vi "Match Initiate Upload Response.vi"(8 "error in":errorcluster, 10 "Frame Data":u8[](array[numeric]), 11 "SDO Transfer in":refnum<class "SDO Transfer.lvclass">) -> (0 "error out":errorcluster, 1 "SDO Result":T1={"Success"=FALSE, "SDO abort code"={"Null"=FALSE, "Value"=0}, "Data"={"Null"=TRUE, "Data"=[]}} {"SDO abort code"."Value" items=["Toggle bit not allowed"=84082688, "SDO protocol timed out"=84148224, "Client/server command specifier not valid or unknown"=84148225, "Invalid block size (block mode only)"=84148226, "Invalid sequence number (block mode only)"=84148227, "CRC error (block mode only)"=84148228, "Out of memory"=84148229, "Attempt to read a write only object"=100728833, "Attempt to write a read only object"=100728834, "Object does not exist in the object dictionary"=100794368, "Object cannot be mapped to the PDO"=100925505, "The number and length of the objects to be mapped would exceed PDO length"=100925506, "General parameter incompatibility reason"=100925507, "General internal incompatibility in the device"=100925511, "Access failed due to an hardware error"=101056512, "Data type does not match, length of service parameter does not match"=101122064, "Data type does not match, length of service parameter too high"=101122066, "Data type does not match, length of service parameter too low"=101122067, "Sub-index does not exist"=101253137, "Invalid value for parameter (download only)"=101253168, "Value of parameter written too high (download only)"=101253169, "Value of parameter written too low (download only)"=101253170, "Maximum value is less than minimum value"=101253174, "Resource not available: SDO connection"=101318691, "General error"=134217728, "Data cannot be transferred or stored to the application"=134217760, "Data cannot be transferred or stored to the application because of local control"=134217761, "Data cannot be transferred or stored to the application because of the present device stable"=134217762, "Object dictionary dynamic generation fails or no object dictionary is present (e.g. object dictionary is generated from file and generation fails because of an file error)"=134217763, "No data available"=134217764]; "Data"."Data" format="%02x"}, 2 "Match":bool, 3 "SDO Transfer out":refnum<class "SDO Transfer.lvclass">)   [LabVIEW 2020, in "CANopen.lvlib" / "SDO Manager.lvlib" / "Upload Transfer.lvclass"]
uses:
  Upload Transfer.lvclass
  SDO Transfer/SDO Transfer.lvclass
  Segmented Upload Transfer/Segmented Upload Transfer.lvclass
  HAL/Source/Interfaces/ICommunicate/ICommunicate.lvclass
  Upload Transfer.lvclass/Upload Transfer.ctl
  D:/git/CANopen-LabVIEW/source/SDO Manager/SDO Manager/SDO Transfer/SDO Transfer.lvclass
  D:/git/CANopen-LabVIEW/source/Response Matcher/IResponse/IMatch Response.lvclass
  D:/git/CANopen-LabVIEW/source/SDO Manager/SDO Manager/Segmented Upload Transfer/Segmented Upload Transfer.lvclass
  SDO Transfer/SDO abort code.ctl
  Typedefs/SDO Result.ctl
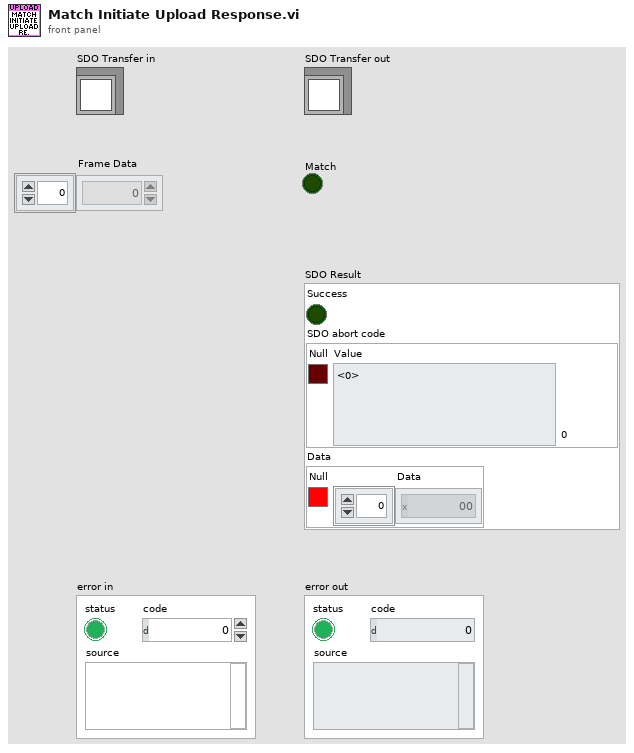
[diagram p1: front panel]
types:
  T1 = typedef "CANopen.lvlib/SDO Manager.lvlib/SDO Transfer.lvclass/SDO Result.ctl" = cluster{"Success":bool, "SDO abort code":cluster{"Null":bool, "Value":T2}, "Data":cluster{"Null":bool, "Data":u8[]}}
  T2 = typedef "CANopen.lvlib/SDO Manager.lvlib/SDO Transfer.lvclass/SDO abort code.ctl" = u32
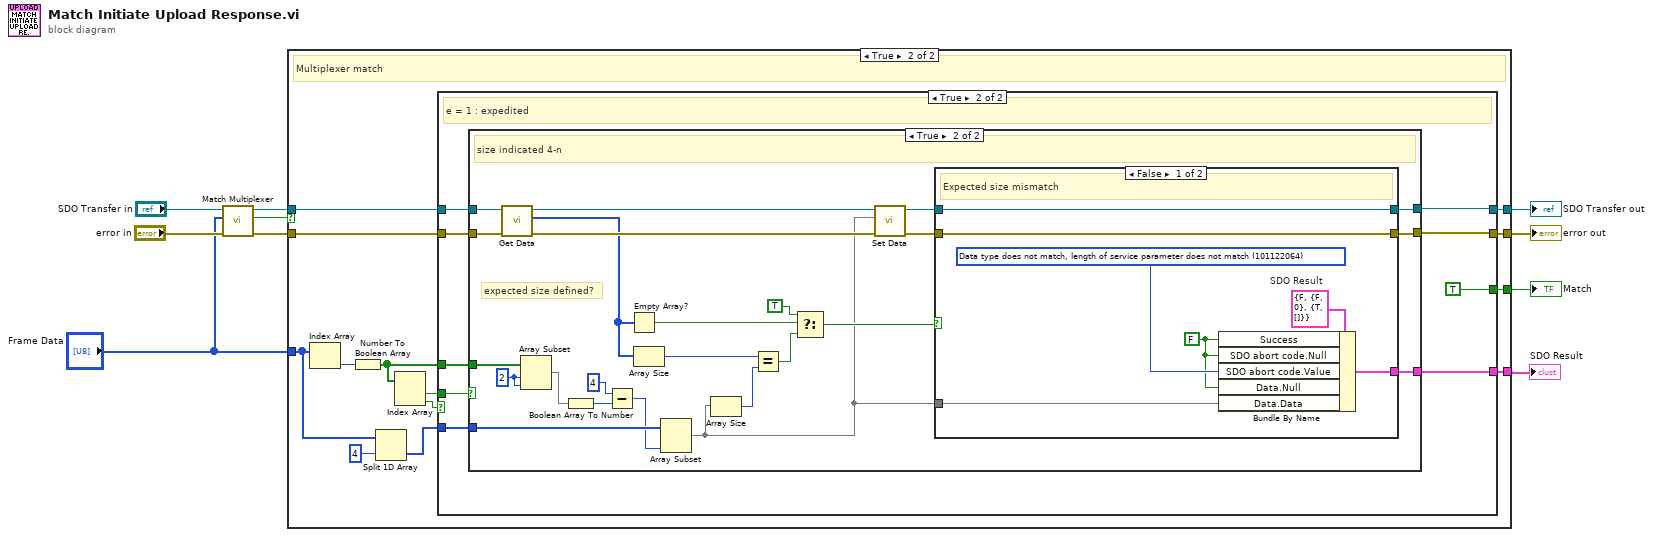
[diagram p0: block diagram]
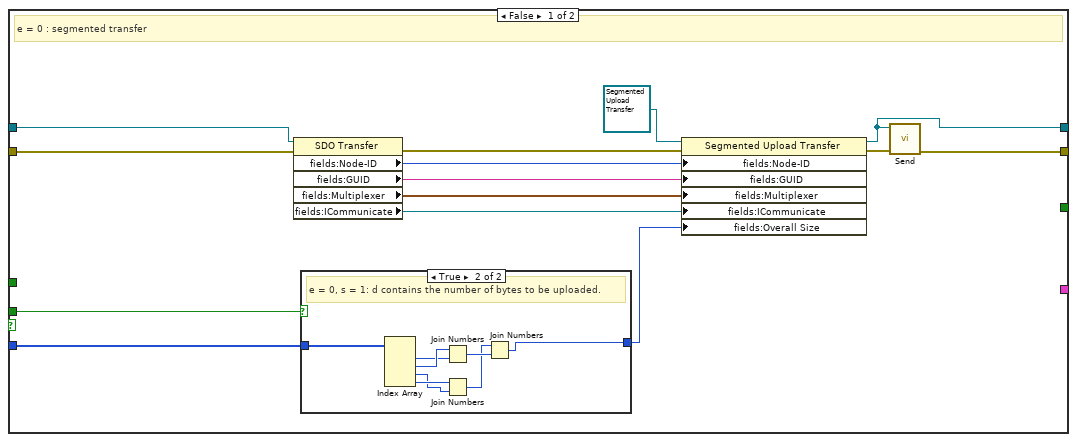
[diagram p3: hidden frame]
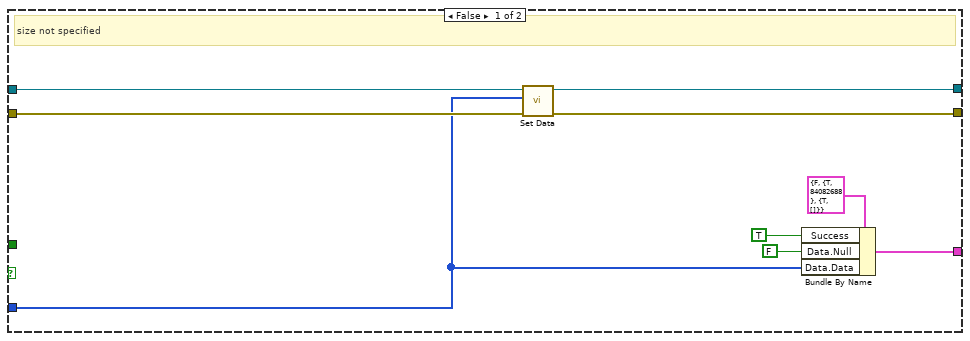
[diagram p5: hidden frame]
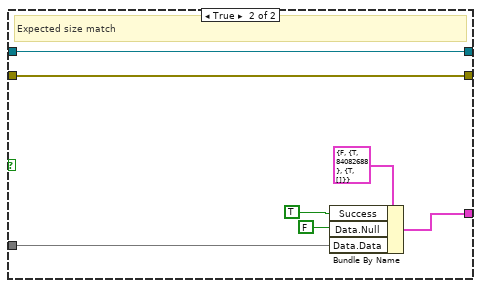
[diagram p6: hidden frame]
diagram:
  n1 = call "Match Multiplexer.vi"("error in"="error in", "Frame Data"="Frame Data", "SDO Transfer in"="SDO Transfer in") -> ("error out"=w5:errorcluster, "Match"=w3:bool, "SDO Transfer out"=w4:refnum<class "SDO Transfer.lvclass">)  [unwired: 6 in]
  n2 = case shown="True" w3 {
    tunnel: [_ w22] -> w10
    tunnel: [w11 w21] -> w9
    tunnel: [w12 w20] -> w7
    tunnel: w5 -> [w12 w19]
    tunnel: w4 -> [w11 w18]
    tunnel: "Frame Data" -> [_ w14]
    tunnel: [_ w13] -> w1
    frame False {
      # "Multiplexer mismatch"
    }
    frame True {
      # "Multiplexer match"
      n3 = Index Array(array=w14) -> (element=w15:u8)  [unwired: 1 in]
      n4 = Number To Boolean Array(number=w15) -> (Boolean array=w23:bool[])
      n5 = Split 1D Array(array=w14, index=4) -> (second subarray=w16:u8[])  [unwired: 1 out]
      n6 = Index Array(array=w23) -> (element #1=w25:bool, element #2=w24:bool)  [unwired: 2 in]
      n7 = case shown="True" w24 {
        tunnel: [w33 w50] -> w20
        tunnel: w18 -> [w39 w52]
        tunnel: [w26 w49] -> w21
        tunnel: [_ TRUE] -> w22
        tunnel: w16 -> [w37 w55]
        tunnel: w25 -> [w38 w54]
        tunnel: w23 -> [_ w53]
        tunnel: w19 -> [w27 w51]
        tunnel: [_ w48] -> w13
        frame False {
          # "e = 0 : segmented transfer"
          n8 = property class="SDO Transfer"(reference=w39, error in=w27) -> (error out=w35:errorcluster, "fields:Node-ID"=w30:u8, "fields:GUID"=w28:string, "fields:Multiplexer"=w31:cluster{"Index":u16, "Sub-Index":u8}, "fields:ICommunicate"=w32:refnum<class "ICommunicate.lvclass">)  [unwired: 1 out]
          n9 = case shown="True" w38 {
            tunnel: w37 -> [_ w47]
            tunnel: [_ w40] -> w29
            frame False {
              # "e = 0, s = 0 d is reserved for further use"
            }
            frame True {
              # "e = 0, s = 1: d contains the number of bytes to be uploaded."
              n10 = Index Array(array=w47) -> (element #1=w43:u8, element #2=w44:u8, element #3=w45:u8, element #4=w46:u8)  [unwired: 4 in]
              n11 = Join Numbers(hi=w44, lo=w43) -> ((hi.lo)=w42:u16)
              n12 = Join Numbers(hi=w46, lo=w45) -> ((hi.lo)=w41:u16)
              n13 = Join Numbers(hi=w41, lo=w42) -> ((hi.lo)=w40:u32)
            }
          }
          n14 = property class="Segmented Upload Transfer"(reference=refnum<class "Segmented Upload Transfer.lvclass"> refnum ("CANopen Master:Segmented Upload Transfer.lvclass"), error in=w35, "fields:Node-ID"=w30, "fields:GUID"=w28, "fields:Multiplexer"=w31, "fields:ICommunicate"=w32, "fields:Overall Size"=w29) -> (reference out=w26:refnum<class "Segmented Upload Transfer.lvclass">, error out=w34:errorcluster)
          n15 = call-dynamic "Send.vi"("error in"=w34, "Segmented Upload Transfer"=w26) -> ("error out"=w33:errorcluster)  [unwired: 9 in]
        }
        frame True {
          # "e = 1 : expedited"
          n16 = case shown="True" w54 {
            tunnel: w55 -> [w57 w89]
            tunnel: w53 -> [_ w86]
            tunnel: w52 -> [w63 w81]
            tunnel: w51 -> [w62 w82]
            tunnel: [w65 w69] -> w50
            tunnel: [w64 w68] -> w49
            tunnel: [w59 w67] -> w48
            frame False {
              # "size not specified"
              n17 = call "Set Data.vi"("error in"=w62, "Data"=w57, "SDO Transfer in"=w63) -> ("error out"=w65:errorcluster, "SDO Transfer out"=w64:refnum<class "SDO Transfer.lvclass">)  [unwired: 7 in]
              n18 = Bundle By Name(cluster=T1 {"Success"=FALSE, "SDO abort code"={"Null"=TRUE, "Value"=84082688}, "Data"={"Null"=TRUE, "Data"=[]}} ("SDO Result"), "Success"=TRUE, "Data.Null"=FALSE, "Data.Data"=w57) -> (w59:T1)
            }
            frame True {
              w85 = 2 ("index")
              # "expected size defined?"
              # "size indicated 4-n"
              n19 = call "Get Data.vi"("error in"=w82, "SDO Transfer in"=w81) -> ("error out"=w80:errorcluster, "Data"=w76:u8[], "SDO Transfer out"=w79:refnum<class "SDO Transfer.lvclass">)  [unwired: 7 in]
              n20 = Array Subset(array=w86, index=w85, length=w85) -> (w83:bool[])
              n21 = Boolean Array To Number(Boolean array=w83) -> (number=w84:u32)
              n22 = Subtract(x=u32 4, y=w84) -> (x-y=w88:u32)
              n23 = Empty Array?(array=w76) -> (empty?=w75:bool)
              n24 = Array Size(array=w76) -> (size(s)=w73:i32)
              n25 = Array Subset(array=w89, length=w88) -> (w66:u8[])  [unwired: 1 in]
              n26 = Array Size(array=w66) -> (size(s)=w74:i32)
              n27 = Equal?(x=w73, y=w74) -> (x = y?=w72:bool)
              n28 = Select(t=TRUE, s=w75, f=w72) -> (s? t:f=w70:bool)
              n29 = call "Set Data.vi"("error in"=w80, "Data"=w66, "SDO Transfer in"=w79) -> ("error out"=w78:errorcluster, "SDO Transfer out"=w77:refnum<class "SDO Transfer.lvclass">)  [unwired: 7 in]
              n30 = case shown="False" w70 {
                tunnel: w78 -> [w92 w103]
                tunnel: w77 -> [w91 w98]
                tunnel: [w92 w103] -> w69
                tunnel: [w91 w98] -> w68
                tunnel: [w94 w101] -> w67
                tunnel: w66 -> [w90 w97]
                frame False {
                  w93 = FALSE ("SDO Result.Success")
                  w96 = T1 {"Success"=FALSE, "SDO abort code"={"Null"=FALSE, "Value"=0}, "Data"={"Null"=TRUE, "Data"=[]}}  # SDO Result
                  w95 = T2 101122064 items=["Toggle bit not allowed"=84082688, "SDO protocol timed out"=84148224, "Client/server command specifier not valid or unknown"=84148225, "Invalid block size (block mode only)"=84148226, "Invalid sequence number (block mode only)"=84148227, "CRC error (block mode only)"=84148228, "Out of memory"=84148229, "Attempt to read a write only object"=100728833, "Attempt to write a read only object"=100728834, "Object does not exist in the object dictionary"=100794368, "Object cannot be mapped to the PDO"=100925505, "The number and length of the objects to be mapped would exceed PDO length"=100925506, "General parameter incompatibility reason"=100925507, "General internal incompatibility in the device"=100925511, "Access failed due to an hardware error"=101056512, "Data type does not match, length of service parameter does not match"=101122064, "Data type does not match, length of service parameter too high"=101122066, "Data type does not match, length of service parameter too low"=101122067, "Sub-index does not exist"=101253137, "Invalid value for parameter (download only)"=101253168, "Value of parameter written too high (download only)"=101253169, "Value of parameter written too low (download only)"=101253170, "Maximum value is less than minimum value"=101253174, "Resource not available: SDO connection"=101318691, "General error"=134217728, "Data cannot be transferred or stored to the application"=134217760, "Data cannot be transferred or stored to the application because of local control"=134217761, "Data cannot be transferred or stored to the application because of the present device stable"=134217762, "Object dictionary dynamic generation fails or no object dictionary is present (e.g. object dictionary is generated from file and generation fails because of an file error)"=134217763, "No data available"=134217764] ("SDO abort code")
                  # "Expected size mismatch"
                  n31 = Bundle By Name(cluster=w96, "Success"=w93, "SDO abort code.Null"=w93, "SDO abort code.Value"=w95, "Data.Null"=w93, "Data.Data"=w90) -> (w94:T1)
                }
                frame True {
                  # "Expected size match"
                  n32 = Bundle By Name(cluster=T1 {"Success"=FALSE, "SDO abort code"={"Null"=TRUE, "Value"=84082688}, "Data"={"Null"=TRUE, "Data"=[]}} ("SDO Result"), "Success"=TRUE, "Data.Null"=FALSE, "Data.Data"=w97) -> (w101:T1)
                }
              }
            }
          }
        }
      }
    }
  }
  "Match" <- w10
  "SDO Transfer out" <- w9
  "error out" <- w7
  "SDO Result" <- w1
